vi "testDataPass_v2,01_vi0.vi"() -> ()   [LabVIEW 2014]
uses:
  testDataPass_v2,0_global1.vi
panel:
  in  "stop":bool
  out "error out 2":errorcluster
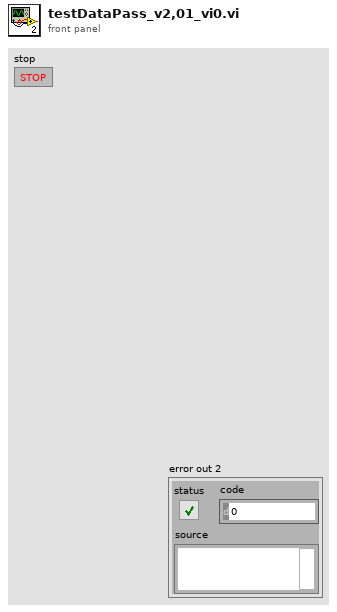
[diagram p1: front panel]
types:
  T1 = enum32{"Invalid", "Standard", "Closed", "Hidden", "Minimized", "Maximized"}
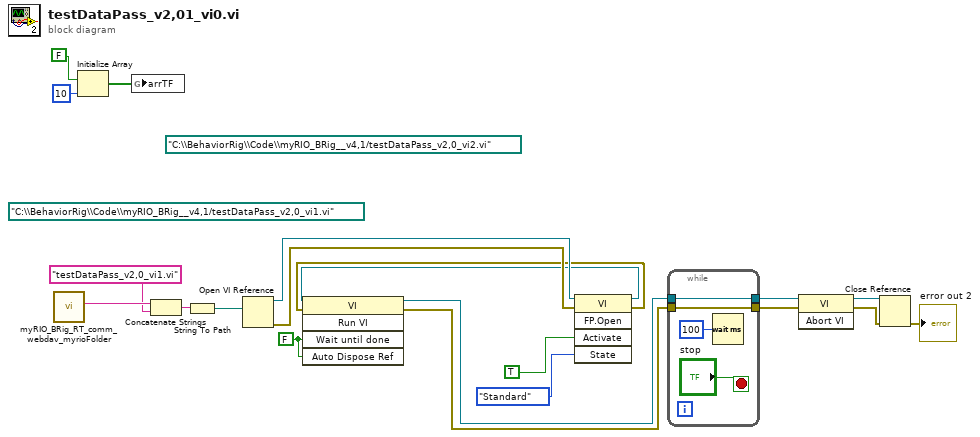
[diagram p0: block diagram]
diagram:
  w7 = FALSE ("Wait Until Done")
  (unwired) path "C:\\BehaviorRig\\Code\\myRIO_BRig__v4,1/testDataPass_v2,0_vi1.vi" ("vi path")
  (unwired) path "C:\\BehaviorRig\\Code\\myRIO_BRig__v4,1/testDataPass_v2,0_vi2.vi" ("vi path")
  n1 = call "myRIO_BRig_RT_comm_webdav_myrioFolder.vi"() -> ("output_myrioFolder"=w21:string)  [unwired: 11 in]
  n2 = Initialize Array(FALSE, 10 ("dimension size")) -> (w19:bool[])
  n3 = global write "testDataPass_v2,0_global1.vi" "arrTF"(w19) -> ()
  n4 = Concatenate Strings(w21, "testDataPass_v2,0_vi1.vi" ("string")) -> (w16:string)
  n5 = String To Path(string=w16) -> (path=w12:path)
  n6 = Open VI Reference(vi path=w12) -> (vi reference=w6:refnum<vi>, error out=w5:errorcluster)  [unwired: 5 in]
  n7 = invoke class="VI" method="FP.Open"(reference=w6, error in=w5, "Activate"=TRUE ("Activate?"), "State"=T1."Standard") -> (reference out=w4:refnum<vi>, error out=w3:errorcluster)  [unwired: 1 in, 3 out]
  n8 = invoke class="VI" method="Run VI"(reference=w4, error in=w3, "Wait until done"=w7, "Auto Dispose Ref"=w7) -> (reference out=w2:refnum<vi>, error out=w1:errorcluster)  [unwired: 1 in, 3 out]
  n9 = while {
    tunnel: w2 -> [w23]
    tunnel: w1 -> [w22]
    tunnel: [w23] -> w11
    tunnel: [w22] -> w10
    stop <- "stop" stop-if-true
    n10 = Wait (ms)(milliseconds to wait=u32 100) -> ()  [unwired: 1 out]
  }
  n11 = invoke class="VI" method="Abort VI"(reference=w11, error in=w10) -> (reference out=w9:refnum<vi>, error out=w8:errorcluster)  [unwired: 1 in, 1 out]
  n12 = Close Reference(reference=w9, error in (no error)=w8) -> (error out=→"error out 2":errorcluster)
